vi "unused_moveBy.vi"(4 "dy(vertical)":i32, 6 "dx(horiziontal)":i32, 8 "error in (no error)":errorcluster, 11 "GObject in":refnum<class "GObject.lvclass">) -> (0 "error out":errorcluster, 3 "GObject out":refnum<class "GObject.lvclass">)   [LabVIEW 2023]
uses:
  GObject.lvclass
  Read position.vi
  Write position.vi
  GObject.lvclass/GObject.ctl
panel:
  # "\\"
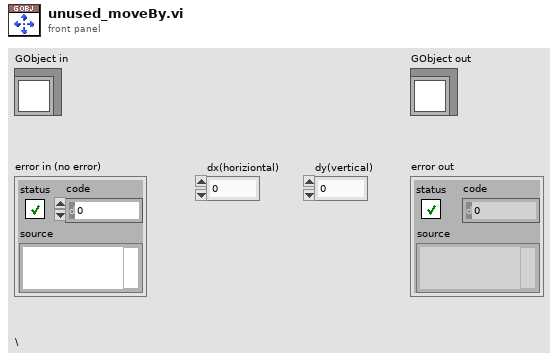
[diagram p1: front panel]
types:
  T1 = typedef "LVPositionTypeDef.ctl" = cluster{"Left":i32, "Top":i32}
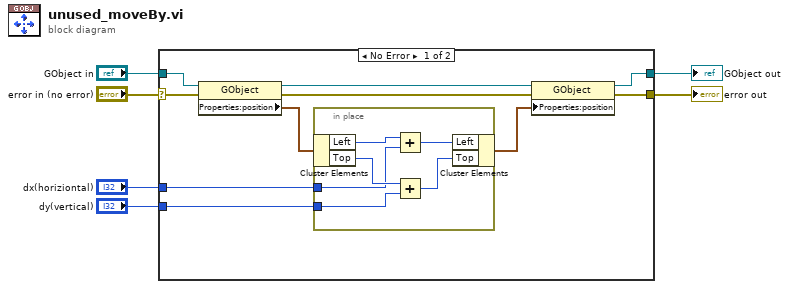
[diagram p0: block diagram]
diagram:
  n1 = case shown="No Error" "error in (no error)" {
    selector: "error in (no error)" -> [w10 w24]
    tunnel: [w9 w24] -> w5
    tunnel: [w15 w23] -> w3
    tunnel: "GObject in" -> [w14 w23]
    tunnel: "dy(vertical)" -> [w8 _]
    tunnel: "dx(horiziontal)" -> [w7 _]
    frame No Error {
      n2 = property class="GObject"(reference=w14, error in=w10) -> (reference out=w16:refnum<class "GObject.lvclass">, error out=w11:errorcluster, "Properties:position"=w13:T1)
      n3 = in-place {
        in-place-border: w8 -> [w19]
        in-place-border: w7 -> [w17]
        n4 = in-place-cluster #1(w13) -> ("Left"=w22:i32, "Top"=w20:i32)
        n5 = Add(x=w22, y=w17) -> (x+y=w21:i32)
        n6 = Add(x=w20, y=w19) -> (x+y=w18:i32)
        n7 = in-place-cluster #1("Left"=w21, "Top"=w18) -> (w12:T1)
      }
      n8 = property class="GObject"(reference=w16, error in=w11, "Properties:position"=w12) -> (reference out=w15:refnum<class "GObject.lvclass">, error out=w9:errorcluster)
    }
    frame Error {
    }
  }
  "error out" <- w5
  "GObject out" <- w3
